vi "getName.vi"(8 "error in (no error)":errorcluster, 11 "RealCustomer in":refnum<class "RealCustomer.lvclass">) -> (0 "error out":errorcluster, 2 "name":string, 3 "RealCustomer out":refnum<class "RealCustomer.lvclass">)   [LabVIEW 2018, in "RealCustomer.lvclass"]
uses:
  RealCustomer.lvclass
  RealCustomer.lvclass/RealCustomer.ctl
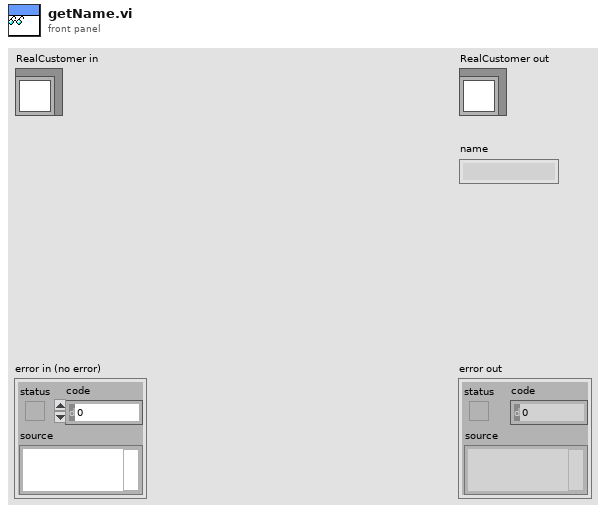
[diagram p1: front panel]
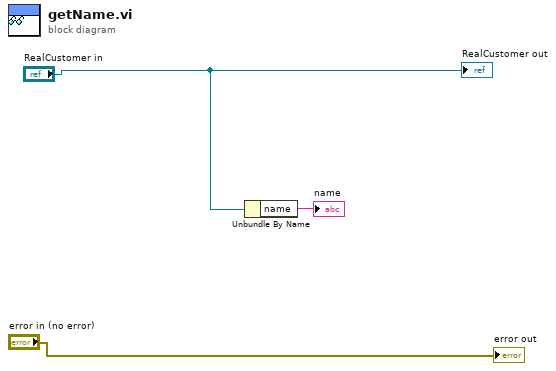
[diagram p0: block diagram]
diagram:
  n1 = Unbundle By Name("RealCustomer in") -> ("name"=→"name":string)
  "error out" <- "error in (no error)"
  "RealCustomer out" <- "RealCustomer in"
